vi "Sound_Acquire_Data_and_Write_to_File_Time_Elapsed.vi"() -> ()   [LabVIEW 2020]
uses:
  <vilib>/sound2/lvsound2.llb/Sampling Mode.ctl
  <vilib>/sound2/lvsound2.llb/Sound Data Format.ctl
  <vilib>/sound2/lvsound2.llb/Sound File Write Open.vi
  <vilib>/sound2/lvsound2.llb/Sound Input Read (DBL).vi
  <vilib>/sound2/lvsound2.llb/Sound File Write (DBL).vi
panel:
  out "Sound Waveform - Channel 2":waveform(dbl)(graph)
  in  "Stop":bool
  out "Reocrd Time":string
  in  "Recording Period [s]":dbl=5.0
  out "Sound Waveform - Channel 1":waveform(dbl)(graph)
  out "WAV File Path":path
  in  "Device ID":u32
  # "Acquire Sound Data and Write to File"
  # "Auther: Suparat Yeamkuan\nOverview: Acquire sound from computer microphone and write to WAV file.\nRequirements: Microphone"
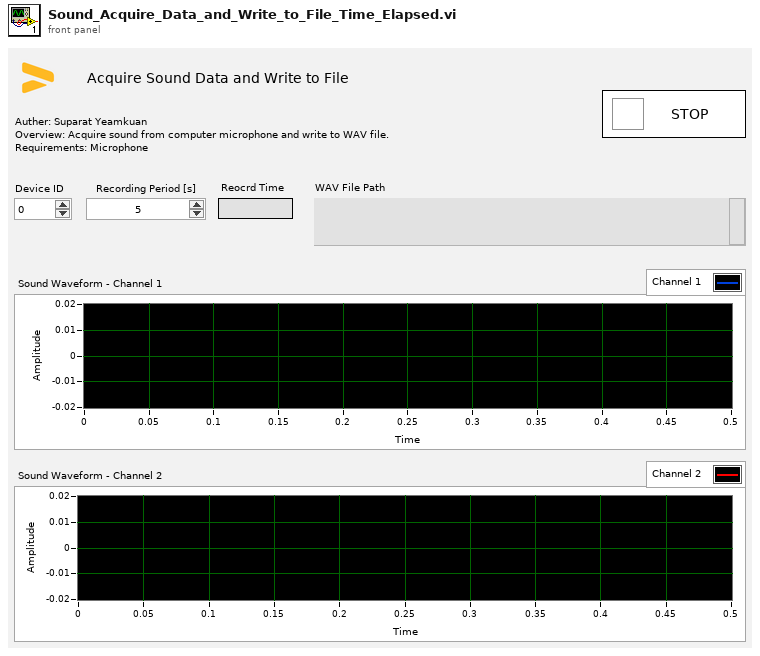
[diagram p1: front panel]
types:
  T1 = typedef "Sound Data Format.ctl" = cluster{"sample rate (S/s)":dbl, "number of channels":i32, "bits per sample":i32}
  T2 = typedef "Sampling Mode.ctl" = i32
  T3 = typedef "Sound File Refnum.ctl" = refnum<file>
  T4 = typedef "Sound Input Task ID.ctl" = u32
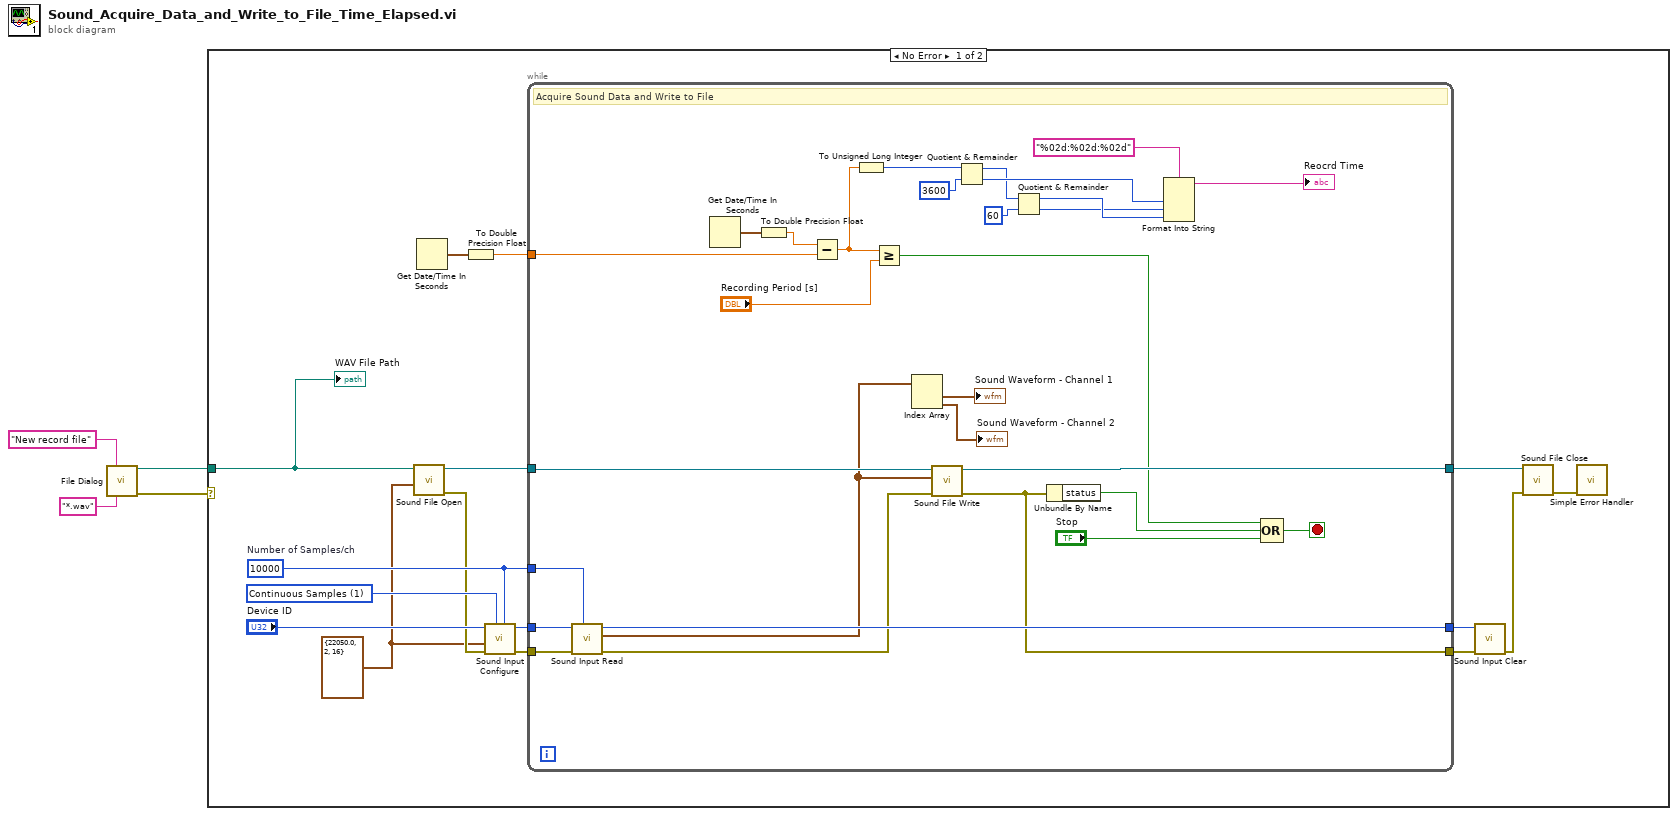
[diagram p0: block diagram]
diagram:
  n1 = call "File Dialog"("prompt"="New record file", "pattern (all files)"="*.wav") -> ("selected path"=w4:path, "error out"=w1:errorcluster)  [unwired: 10 in, 2 out]
  n2 = case shown="No Error" w1 {
    tunnel: w4 -> [w5 _]
    frame No Error {
      w8 = T1 {"sample rate (S/s)"=22050.0, "number of channels"=2, "bits per sample"=16} ("Sound Format")
      w15 = 10000  # Number of Samples/ch
      w14 = T2 1 items=["Finite Samples", "Continuous Samples"] ("sample mode")
      n3 = call-poly <vilib>:"Sound File Open.vi"("sound format"=w8, "path"=w5) -> ("error out"=w10:errorcluster, "sound file refnum"=w13:T3)  [unwired: 8 in]
      n4 = Get Date/Time In Seconds() -> (seconds since 1Jan1904=w7:timestamp)
      n5 = To Double Precision Float(number=w7) -> (double precision float=w6:dbl)
      n6 = call <vilib>:"Sound Input Configure.vi"("number of samples/ch"=w15, "sample mode"=w14, "error in (no error)"=w10, "sound format"=w8, "device ID"="Device ID") -> ("error out"=w20:errorcluster, "task ID"=w18:T4)  [unwired: 5 in]
      n7 = while {
        tunnel: w15 -> [w46]
        tunnel: w13 -> [w44]
        tunnel: [w43] -> w12
        tunnel: w18 -> [w48]
        tunnel: [w47] -> w17
        tunnel: w20 -> [w49]
        tunnel: [w37] -> w16
        tunnel: w6 -> [w38]
        stop <- w45 stop-if-true
        # "Acquire Sound Data and Write to File"
        n8 = call-poly <vilib>:"Sound Input Read.vi"("number of samples/ch"=w46, "error in (no error)"=w49, "task ID"=w48) -> ("error out"=w42:errorcluster, "data"=w33:waveform(dbl)[], "task ID out"=w47:T4)  [unwired: 6 in]
        n9 = Get Date/Time In Seconds() -> (seconds since 1Jan1904=w41:timestamp)
        n10 = To Double Precision Float(number=w41) -> (double precision float=w40:dbl)
        n11 = Subtract(x=w40, y=w38) -> (x-y=w22:dbl)
        n12 = To Unsigned Long Integer(number=w22) -> (unsigned 32bit integer=w29:u32)
        n13 = Greater Or Equal?(x=w22, y="Recording Period [s]") -> (x >= y?=w35:bool)
        n14 = Index Array(array=w33) -> (element #1=→"Sound Waveform - Channel 1":waveform(dbl), element #2=→"Sound Waveform - Channel 2":waveform(dbl))  [unwired: 2 in]
        n15 = call-poly <vilib>:"Sound File Write.vi"("error in (no error)"=w42, "data"=w33, "sound file refnum"=w44) -> ("error out"=w37:errorcluster, "sound file refnum out"=w43:T3)  [unwired: 7 in]
        n16 = Quotient & Remainder(x=w29, y=u32 3600) -> (x-y*floor(x/y)=w25:u32, floor(x/y)=w27:u32)
        n17 = Quotient & Remainder(x=w25, y=u32 60) -> (x-y*floor(x/y)=w30:u32, floor(x/y)=w28:u32)
        n18 = Unbundle By Name(w37) -> ("status"=w36:bool)
        n19 = Format Into String(format string="%02d:%02d:%02d" ("String Format"), w27, w28, w30) -> (resulting string=→"Reocrd Time":string)  [unwired: 2 in, 1 out]
        n20 = Compound Arithmetic op=OR(w35, w36, "Stop") -> (w45:bool)
      }
      n21 = call <vilib>:"Sound Input Clear.vi"("error in (no error)"=w16, "task ID"=w17) -> ("error out"=w11:errorcluster)  [unwired: 9 in]
      n22 = call <vilib>:"Sound File Close.vi"("error in (no error)"=w11, "sound file refnum"=w12) -> ("error out"=w9:errorcluster)  [unwired: 9 in]
      n23 = call <vilib>:"Simple Error Handler.vi"("error in (no error)"=w9) -> ()  [unwired: 4 in, 5 out]
      "WAV File Path" <- w5
    }
    frame Error {
    }
  }
